vi "状态告警区_正常.vi"(11 "数组":u16[](array[numeric]) format="%04xH") -> (2 "状态告警区 2":T1 {"工作状态" items=["空闲"=0, "水样测试"=1, "标样核查"=2, "零点核查"=3, "跨度核查"=4, "空白测试"=5, "平行样测试"=6, "加标回收"=7, "空白校准"=8, "标样校准"=9, "初始化（清洗）"=10, "单步调试"=254, "简易步骤"=255]; "告警代码" items=["无告警", "缺试剂告警", "缺水样告警", "缺蒸馏水告警", "缺标液告警", "仪表漏液告警", "标定异常告警", "超量程告警", "加热异常", "低试剂预警", "超上限告警", "超下限告警", "仪表内部其他异常", "滴定异常告警", "电极异常告警", "量程切换告警", "参数设置告警", "PH电极电位异常", "电导率电极异常", "浊度光度异常", "溶解氧电极异常", "溶解氧光强异常", "温度异常告警", "PH异常告警", "溶解氧异常告警", "电导率异常告警", "浊度异常告警", "叶绿素异常告警", "藻密度异常告警", "蓝绿藻异常告警", "ORP异常告警", "氨氮异常告警", "清洁刷异常告警", "SD卡异常告警", "蓝牙异常告警", "Wifi异常告警", "流程异常告警"]; "故障代码" items=["无故障", "电机故障", "温度故障", "通讯故障", "滴定故障"]}, 3 "状态告警区":T2 {"工作状态" items=["空闲"=0, "水样测试"=1, "标样核查"=2, "零点核查"=3, "跨度核查"=4, "空白测试"=5, "平行样测试"=6, "加标回收"=7, "空白校准"=8, "标样校准"=9, "初始化（清洗）"=10, "单步调试"=254, "简易步骤"=255]; "告警代码" items=["无告警", "缺试剂告警", "缺水样告警", "缺蒸馏水告警", "缺标液告警", "仪表漏液告警", "标定异常告警", "超量程告警", "加热异常", "低试剂预警", "超上限告警", "超下限告警", "仪表内部其他异常", "滴定异常告警", "电极异常告警", "量程切换告警", "参数设置告警", "PH电极电位异常", "电导率电极异常", "浊度光度异常", "溶解氧电极异常", "溶解氧光强异常", "温度异常告警", "PH异常告警", "溶解氧异常告警", "电导率异常告警", "浊度异常告警", "叶绿素异常告警", "藻密度异常告警", "蓝绿藻异常告警", "ORP异常告警", "氨氮异常告警", "清洁刷异常告警", "SD卡异常告警", "蓝牙异常告警", "Wifi异常告警", "流程异常告警"]; "故障代码" items=["无故障", "电机故障", "温度故障", "通讯故障", "滴定故障"]})   [LabVIEW 2016, in "斯坦道总磷总氮.lvlib"]
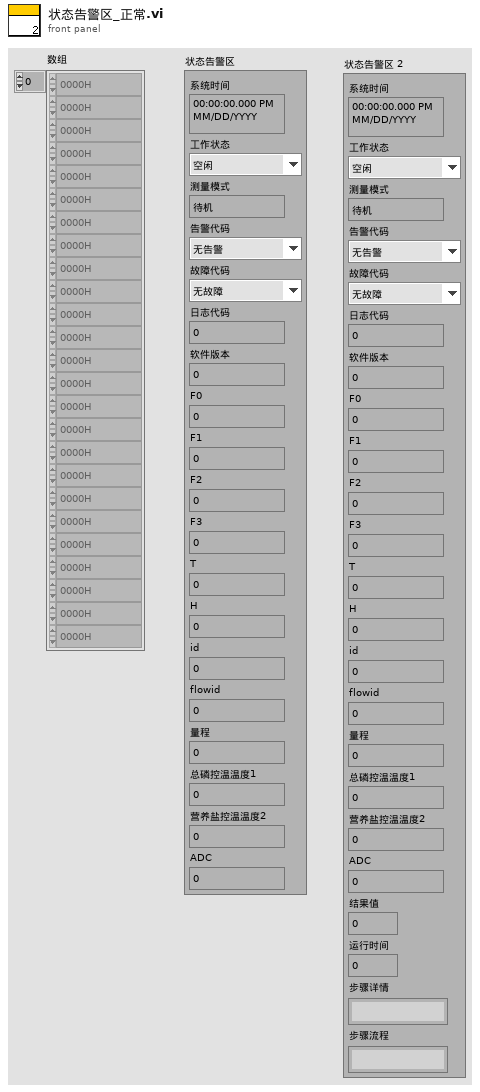
[diagram p1: front panel]
types:
  T1 = cluster{"系统时间":timestamp, "工作状态":u16, "测量模式":enum16{"待机", "连续模式", "周期模式", "定点模式", "受控模式", "手动模式"}, "告警代码":u16, "故障代码":u16, "日志代码":u16, "软件版本":u16, "F0":sgl, "F1":sgl, "F2":sgl, "F3":sgl, "T":sgl, "H":sgl, "id":u16, "flowid":u16, "量程":u16, "总磷控温温度1":sgl, "营养盐控温温度2":sgl, "ADC":sgl, "结果值":sgl, "运行时间":u16, "步骤详情":string, "步骤流程":string}
  T2 = cluster{"系统时间":timestamp, "工作状态":u16, "测量模式":enum16{"待机", "连续模式", "周期模式", "定点模式", "受控模式", "手动模式"}, "告警代码":u16, "故障代码":u16, "日志代码":u16, "软件版本":u16, "F0":sgl, "F1":sgl, "F2":sgl, "F3":sgl, "T":sgl, "H":sgl, "id":u16, "flowid":u16, "量程":u16, "总磷控温温度1":sgl, "营养盐控温温度2":sgl, "ADC":sgl}
  T3 = enum16{"待机", "连续模式", "周期模式", "定点模式", "受控模式", "手动模式"}
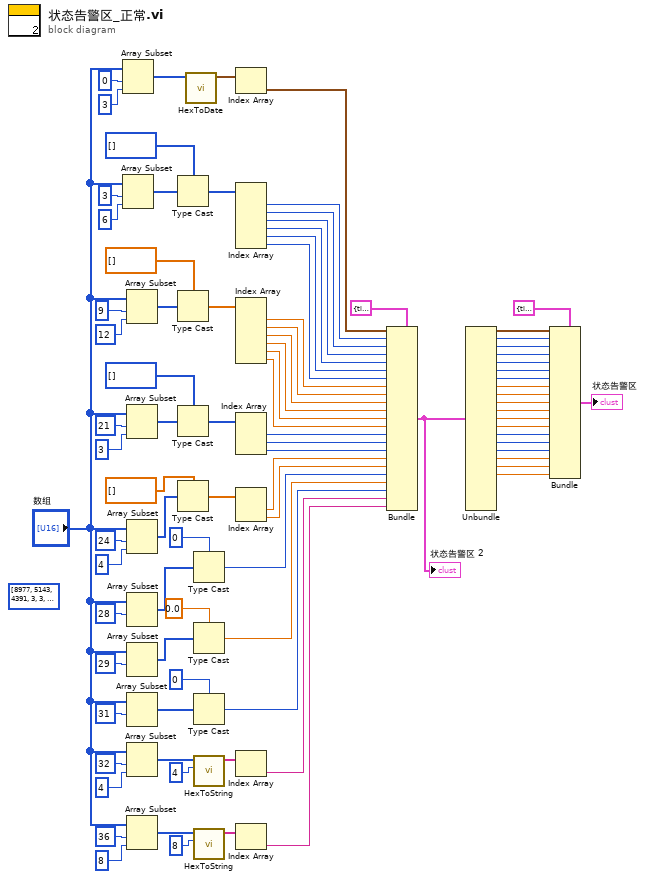
[diagram p0: block diagram]
diagram:
  (unwired) u32[] [8977, 5143, 4391, 3, 3, 0, 0, 45, 0, 9999, 9999, 9999, 9999, 0, 0, 0, 0, 0, 0, 0, 0, 0, 0, 0, 0, 0, 0, 0, 0, 0, 0, 0, 3, 50, 6, 0, 0, 0, 16384, 34820, 16322, 5088, 48327, 8976, 10605] ("数组")
  n1 = Array Subset(array="数组", index=0 ("索引"), length=3 ("长度")) -> (w88:u16[])
  n2 = Array Subset(array="数组", index=3 ("索引"), length=6 ("长度")) -> (w22:u16[])
  n3 = Array Subset(array="数组", index=9 ("索引"), length=12 ("长度")) -> (w18:u16[])
  n4 = Array Subset(array="数组", index=21 ("索引"), length=3 ("索引")) -> (w15:u16[])
  n5 = Array Subset(array="数组", index=24 ("索引"), length=4 ("索引")) -> (w9:u16[])
  n6 = Array Subset(array="数组", index=28 ("索引")) -> (w12:u16[])  [unwired: 1 in]
  n7 = Array Subset(array="数组", index=29 ("索引")) -> (w7:u16[])  [unwired: 1 in]
  n8 = Array Subset(array="数组", index=31 ("索引")) -> (w3:u16[])  [unwired: 1 in]
  n9 = Array Subset(array="数组", index=32 ("索引"), length=4 ("长度")) -> (w33:u16[])
  n10 = Array Subset(array="数组", index=36 ("索引"), length=8 ("长度")) -> (w25:u16[])
  n11 = Type Cast(type=u16[] [], x=w22) -> (*(type *) &x=w20:u16[])
  n12 = Type Cast(type=sgl[] [], x=w18) -> (*(type *) &x=w17:sgl[])
  n13 = Type Cast(type=u16[] [], x=w15) -> (*(type *) &x=w14:u16[])
  n14 = Type Cast(type=sgl[] [], x=w9) -> (*(type *) &x=w8:sgl[])
  n15 = call "HexToDate.vi"("数组"=w88) -> ("DATE"=w85:timestamp[])  [unwired: 10 in]
  n16 = Type Cast(type=u16 0, x=w12) -> (*(type *) &x=w11:u16)
  n17 = Type Cast(type=sgl 0.0, x=w7) -> (*(type *) &x=w5:sgl)
  n18 = Type Cast(type=u16 0, x=w3) -> (*(type *) &x=w2:u16)
  n19 = call "HexToString.vi"("字符个数"=4, "数组"=w33) -> ("STRING"=w31:string[])  [unwired: 9 in]
  n20 = call "HexToString.vi"("字符个数"=8, "数组"=w25) -> ("STRING"=w27:string[])  [unwired: 9 in]
  n21 = Index Array(array=w85) -> (element=w84:timestamp)  [unwired: 1 in]
  n22 = Index Array(array=w20) -> (element #1=w83:u16, element #2=w82:u16, element #3=w81:u16, element #4=w80:u16, element #5=w79:u16, element #6=w78:u16)  [unwired: 6 in]
  n23 = Index Array(array=w17) -> (element #1=w75:sgl, element #2=w74:sgl, element #3=w73:sgl, element #4=w72:sgl, element #5=w71:sgl, element #6=w70:sgl)  [unwired: 6 in]
  n24 = Index Array(array=w14) -> (element #1=w67:u16, element #2=w66:u16, element #3=w65:u16)  [unwired: 3 in]
  n25 = Index Array(array=w8) -> (element #1=w62:sgl, element #2=w61:sgl)  [unwired: 2 in]
  n26 = Index Array(array=w31) -> (element=w30:string)  [unwired: 1 in]
  n27 = Index Array(array=w27) -> (element=w23:string)  [unwired: 1 in]
  n28 = Bundle(cluster=T1 {"系统时间"=timestamp(0 s since 1904-01-01), "工作状态"=0, "测量模式"=enum."待机", "告警代码"=0, "故障代码"=0, "日志代码"=0, "软件版本"=0, "F0"=0.0, "F1"=0.0, "F2"=0.0, "F3"=0.0, "T"=0.0, "H"=0.0, "id"=0, "flowid"=0, "量程"=0, "总磷控温温度1"=0.0, "营养盐控温温度2"=0.0, "ADC"=0.0, "结果值"=0.0, "运行时间"=0, "步骤详情"="", "步骤流程"=""} ("状态告警区 2"), "系统时间"=w84, "工作状态"=w83, "测量模式"=w82, "告警代码"=w81, "故障代码"=w80, "日志代码"=w79, "软件版本"=w78, "F0"=w75, "F1"=w74, "F2"=w73, "F3"=w72, "T"=w71, "H"=w70, "id"=w67, "flowid"=w66, "量程"=w65, "总磷控温温度1"=w62, "营养盐控温温度2"=w61, "ADC"=w11, "结果值"=w5, "运行时间"=w2, "步骤详情"=w30, "步骤流程"=w23) -> (w58:T1)
  "状态告警区 2" <- w58
  n29 = Unbundle(w58) -> ("系统时间"=w56:timestamp, "工作状态"=w55:u16, "测量模式"=w54:T3, "告警代码"=w53:u16, "故障代码"=w52:u16, "日志代码"=w51:u16, "软件版本"=w50:u16, "F0"=w49:sgl, "F1"=w48:sgl, "F2"=w47:sgl, "F3"=w46:sgl, "T"=w45:sgl, "H"=w44:sgl, "id"=w43:u16, "flowid"=w42:u16, "量程"=w41:u16, "总磷控温温度1"=w40:sgl, "营养盐控温温度2"=w39:sgl, "ADC"=w38:sgl)  [unwired: 4 out]
  n30 = Bundle(cluster=T2 {"系统时间"=timestamp(0 s since 1904-01-01), "工作状态"=0, "测量模式"=enum."待机", "告警代码"=0, "故障代码"=0, "日志代码"=0, "软件版本"=0, "F0"=0.0, "F1"=0.0, "F2"=0.0, "F3"=0.0, "T"=0.0, "H"=0.0, "id"=0, "flowid"=0, "量程"=0, "总磷控温温度1"=0.0, "营养盐控温温度2"=0.0, "ADC"=0.0} ("状态告警区"), "系统时间"=w56, "工作状态"=w55, "测量模式"=w54, "告警代码"=w53, "故障代码"=w52, "日志代码"=w51, "软件版本"=w50, "F0"=w49, "F1"=w48, "F2"=w47, "F3"=w46, "T"=w45, "H"=w44, "id"=w43, "flowid"=w42, "量程"=w41, "总磷控温温度1"=w40, "营养盐控温温度2"=w39, "ADC"=w38) -> (→"状态告警区":T2)
